vi "Get Key Value (RAW).vi"(5 "Key name":string, 6 "Default":string, 7 "Section name":string, 8 "error in (no error)":errorcluster, 11 "Carya Config in":refnum<class "Carya Config.lvclass">) -> (0 "error out":errorcluster, 1 "Found?":bool, 2 "Value":string, 3 "Carya Config out":refnum<class "Carya Config.lvclass">)   [LabVIEW 2013, in "Carya Config.lvclass"]
doc: "Copyright 2018, Carya Automatisering, Wiebe Walstra."
uses:
  Carya Config.lvclass
  CConfig Object/Data.ctl
  CConfig Object/Step In Query/Step In Query.lvclass
  CConfig Object/Add Results Query/Add Results Query.lvclass
  CConfig Object/CConfig Object.lvclass
  CConfig Object/Loop Query/Match Query/Match Query.lvclass
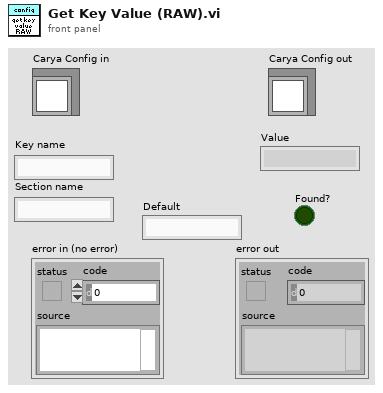
[diagram p1: front panel]
types:
  T1 = typedef "CConfig Object.lvclass/Data.ctl" = enum16{"pre", "name", "middle", "value", "post", "newline", "persistant", "tagged", "type"}
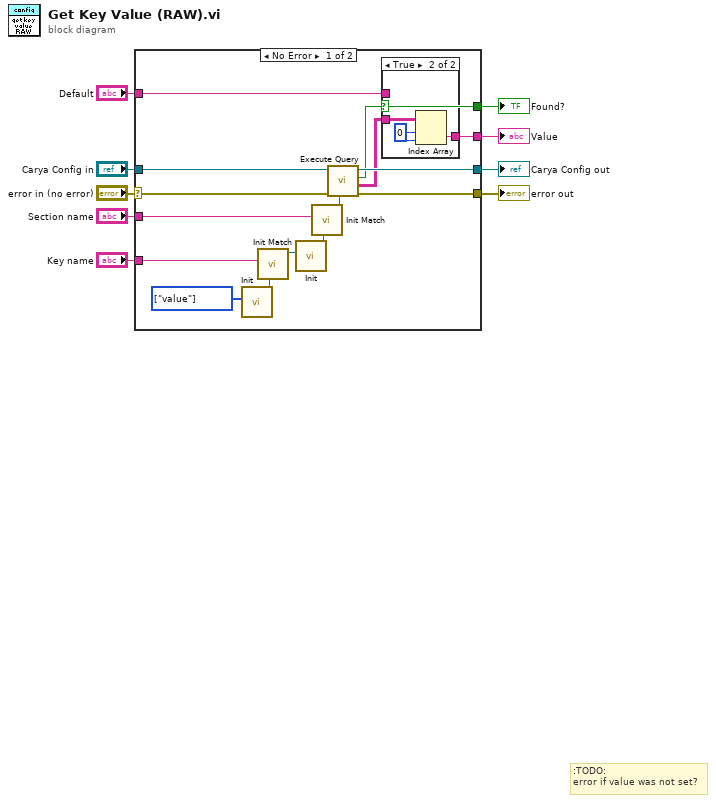
[diagram p0: block diagram]
diagram:
  # ":TODO:\nerror if value was not set?"
  n1 = case shown="No Error" "error in (no error)" {
    selector: "error in (no error)" -> [w20 w31]
    tunnel: [w23 w31] -> w8
    tunnel: [w18 w30] -> w6
    tunnel: "Carya Config in" -> [w19 w30]
    tunnel: "Section name" -> [w24 _]
    tunnel: "Key name" -> [w22 _]
    tunnel: [w11 _] -> w5
    tunnel: [w21 w29] -> w3
    tunnel: "Default" -> [w10 w29]
    frame No Error {
      w17 = T1[] [enum."value"] items=["pre", "name", "middle", "value", "post", "newline", "persistant", "tagged", "type"] ("Data")
      n2 = call "Init.vi"("Data [name]"=w17) -> ("Find First Query out"=w15:refnum<class "Add Results Query.lvclass">)  [unwired: 9 in, 1 out]
      n3 = call "Init Match.vi"("Found"=w15, "Data"=w22) -> ("Find First Query out"=w12:refnum<class "Loop Query.lvclass">)  [unwired: 8 in, 1 out]
      n4 = call "Init.vi"("Config Query"=w12) -> ("Step In Query out"=w14:refnum<class "Step In Query.lvclass">)  [unwired: 9 in, 1 out]
      n5 = call "Init Match.vi"("Found"=w14, "Data"=w24) -> ("Find First Query out"=w13:refnum<class "Loop Query.lvclass">)  [unwired: 8 in, 1 out]
      n6 = call-dynamic "Execute Query.vi"("Config Query in"=w13, "error in (no error)"=w20, "Carya Config in"=w19) -> ("error out"=w23:errorcluster, "Results"=w16:string[][], "Result"=w11:bool, "Carya Config out"=w18:refnum<class "Carya Config.lvclass">)  [unwired: 4 in, 1 out]
      n7 = case shown="True" w11 {
        tunnel: [w25 w28] -> w21
        tunnel: w16 -> [_ w27]
        tunnel: w10 -> [w25 _]
        frame False {
        }
        frame True {
          w26 = 0 ("index (row)")
          n8 = Index Array(array=w27, index (row)=w26, index (col)=w26) -> (element=w28:string)
        }
      }
    }
    frame Error {
    }
  }
  "error out" <- w8
  "Carya Config out" <- w6
  "Found?" <- w5
  "Value" <- w3
